vi "main.vi"() -> ()   [LabVIEW 2014]
uses:
  <vilib>/picture/3D Picture Control/Object/Create Object (drawable).vi
  <vilib>/picture/3D Picture Control/Object/Add Object (reference).vi
  <vilib>/Instr/_visa.llb/VISA Configure Serial Port (Instr).vi
  <vilib>/picture/3D Picture Control/NI_3D Picture Control.lvlib
panel:
  out "8号温度":i32
  out "7号温度":i32
  out "6号温度":i32
  out "未安装":dbl(slide) scale=0.0..5000.0
  out "未安装":dbl(slide) scale=0.0..5000.0
  out "6号温度":dbl(slide) scale=0.0..5000.0
  out "5号温度":dbl(slide) scale=0.0..5000.0
  out "4号温度":dbl(slide) scale=0.0..5000.0
  out "3号温度":dbl(slide) scale=0.0..5000.0
  out "2号温度":dbl(slide) scale=0.0..5000.0
  out "1号温度":dbl(slide) scale=0.0..5000.0
  out "?":T1(graph)
  out "5号温度":i32
  out "4号温度":i32
  out "2号温度":i32
  out "3号温度":i32
  out "1号温度":i32
  in  "停止":bool
  in  "打开":bool caption="stop"
  in  "校验位：":u16(ring) items=["  无校验", "  奇校验", "  偶校验"]
  in  "波特率：":u16(ring)=11 items=["   300", "   600", "   1200", "   2400", "   4800   ", "   9600", "   19200", "   38400", "   43000", "   56000", "   57600", "   115200"]
  in  "通讯口：":u16(ring) items=["   com1", "   com2", "   com3", "   com4", "   com5"]
  out "工作指示灯":bool
  # "TETRAELC--检测DEMO"
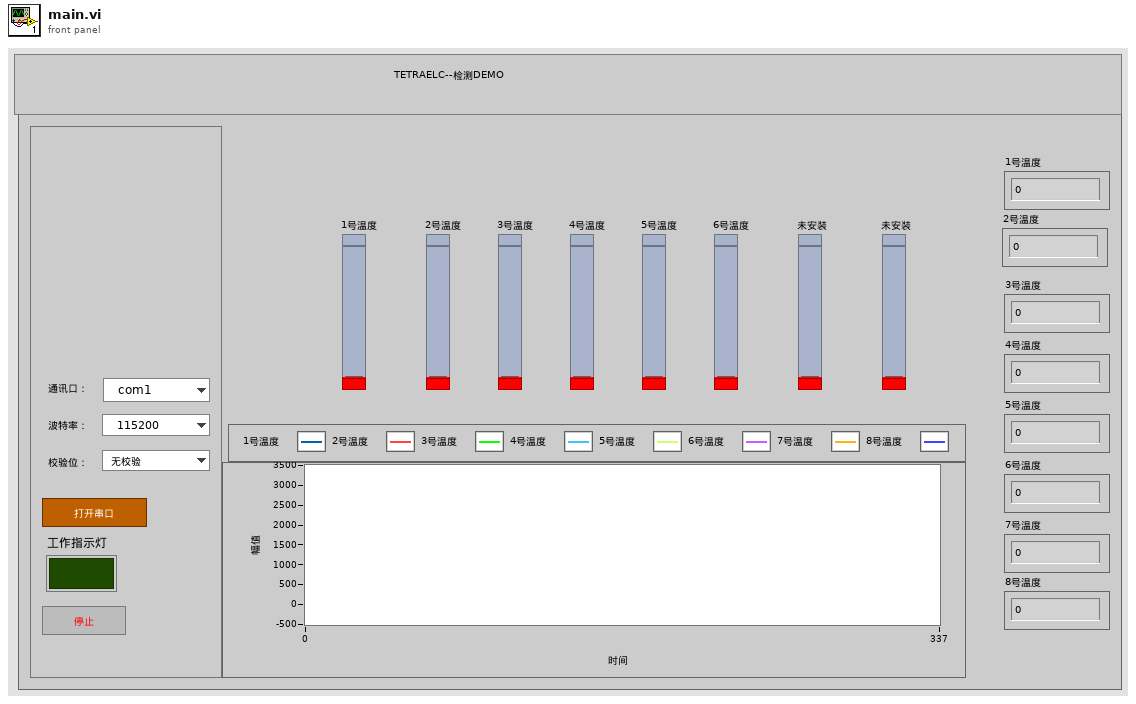
[diagram p1: front panel]
types:
  T1 = cluster{"1号温度":i32, "2号温度":i32, "3号温度":i32, "4号温度":i32, "5号温度":i32, "6号温度":i32, "7号温度":i32, "8号温度":i32}
  T2 = cluster{"T1":i16, "T2":i16, "T3":i16, "T4":i16, "T5":i16, "T6":i16, "T7":i16, "T8":i16}
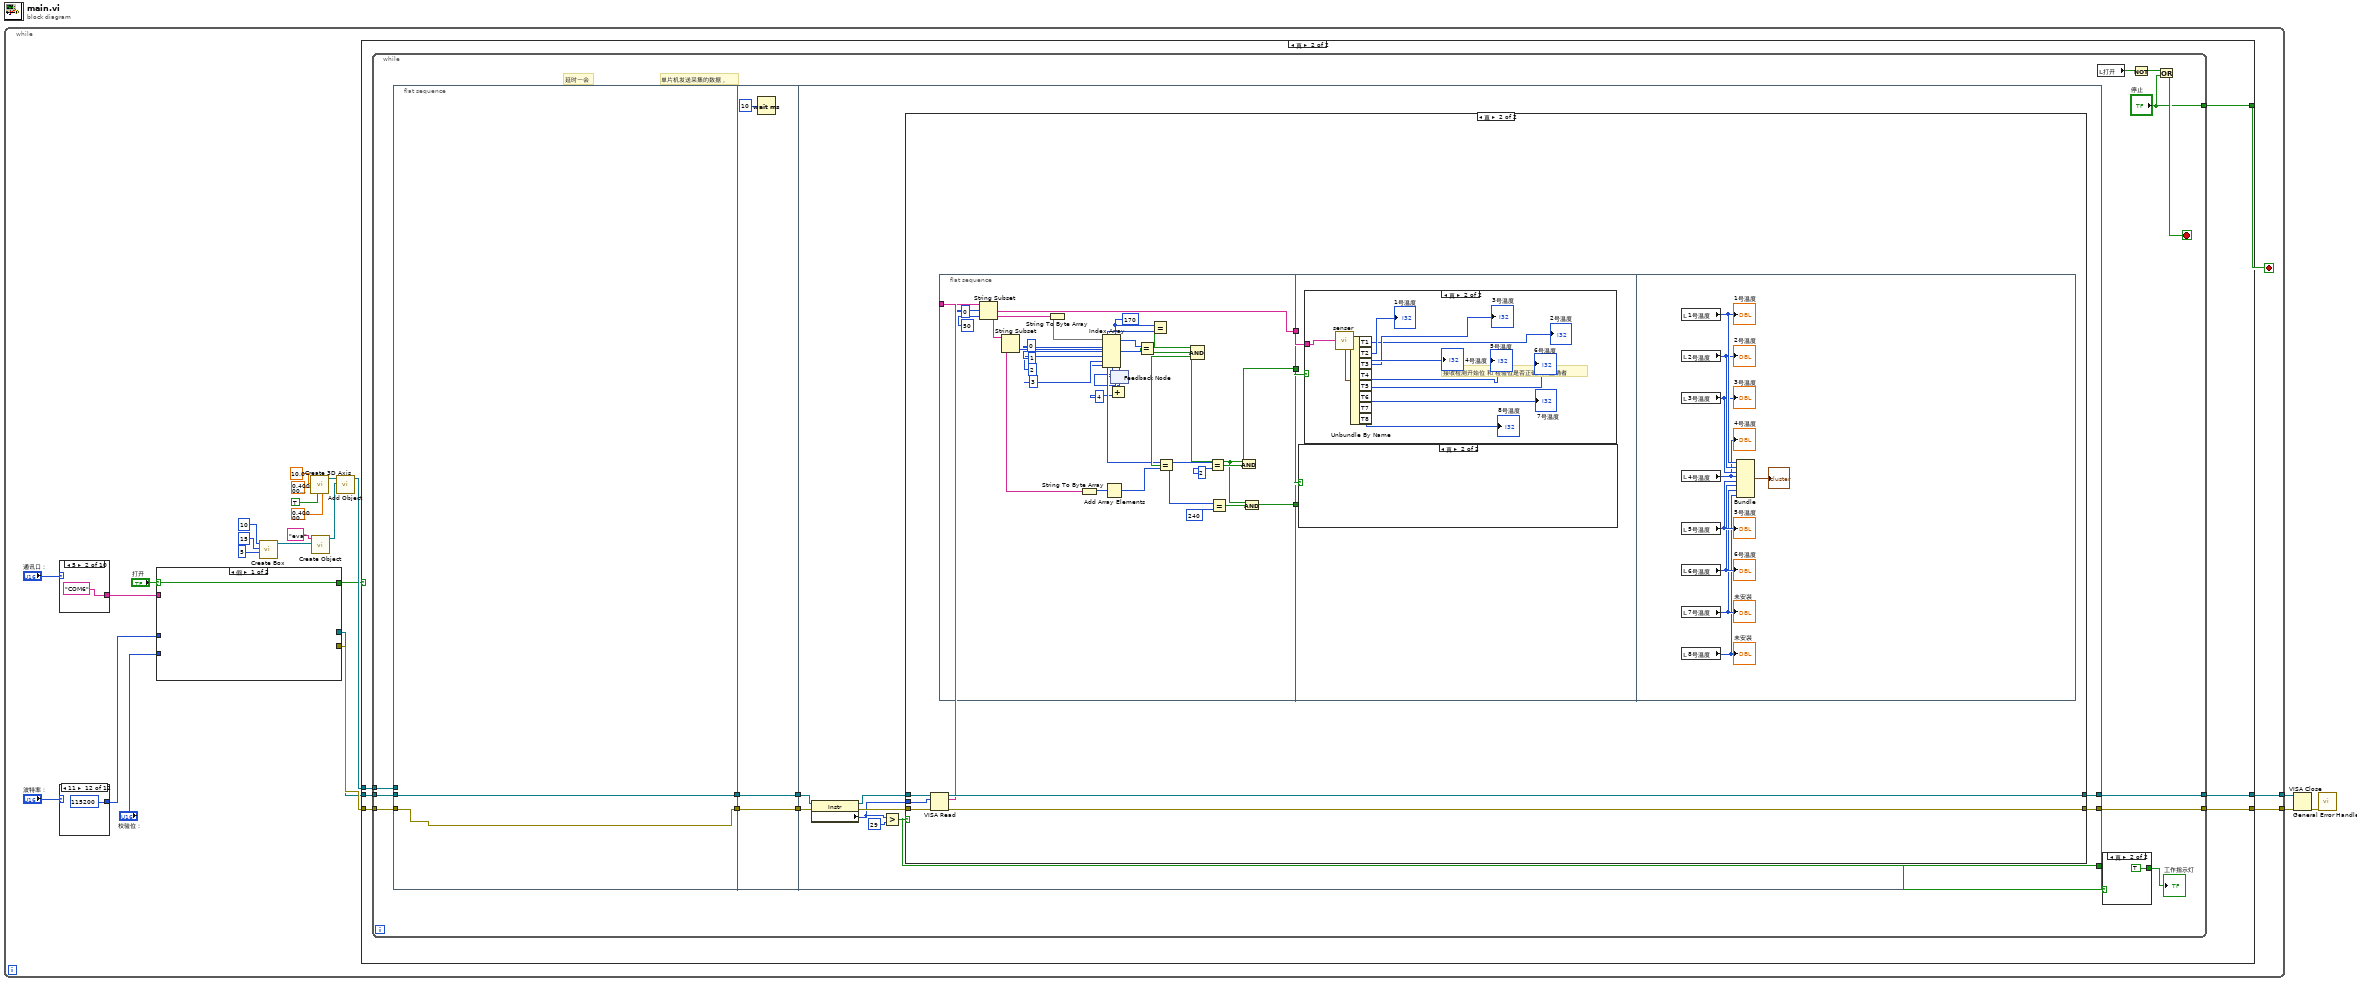
[diagram p0: block diagram]
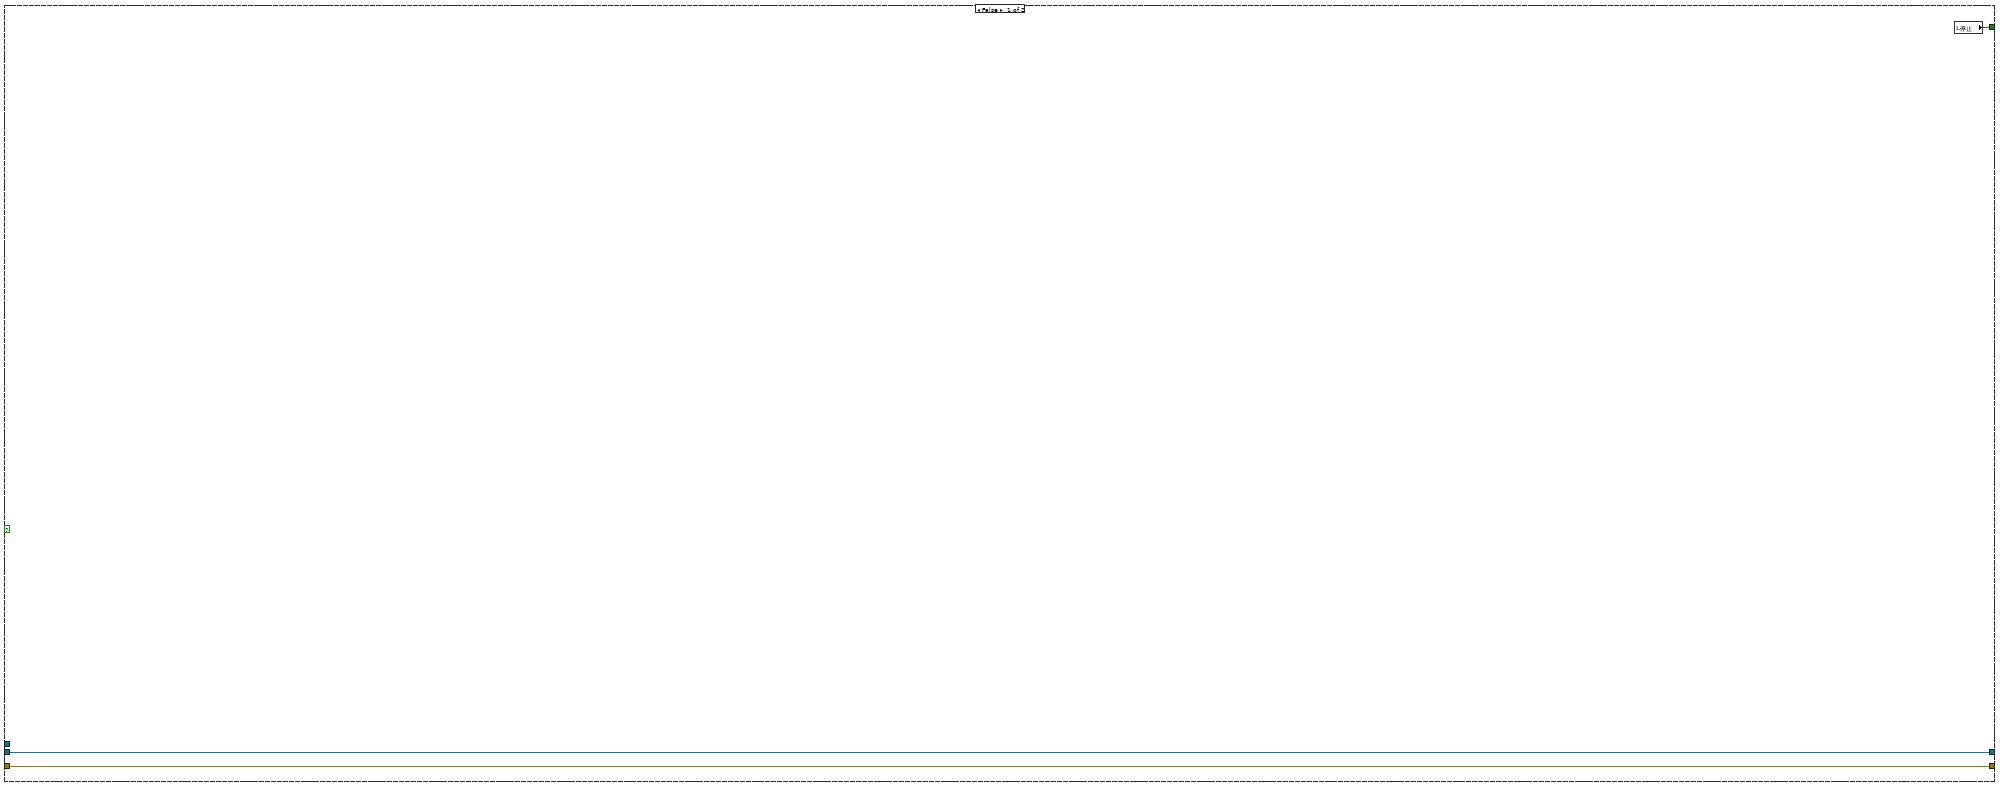
[diagram p2: hidden frame]
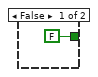
[diagram p3: hidden frame]
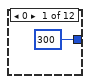
[diagram p7: hidden frame]
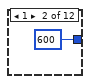
[diagram p8: hidden frame]
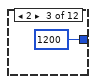
[diagram p9: hidden frame]
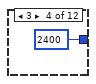
[diagram p10: hidden frame]
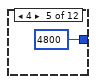
[diagram p11: hidden frame]
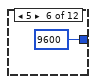
[diagram p12: hidden frame]
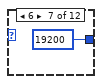
[diagram p13: hidden frame]
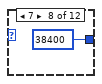
[diagram p14: hidden frame]
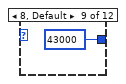
[diagram p15: hidden frame]
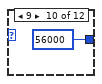
[diagram p16: hidden frame]
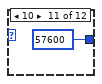
[diagram p17: hidden frame]
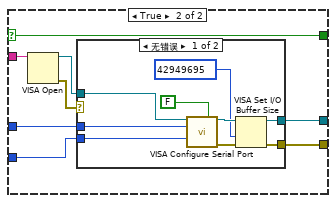
[diagram p18: hidden frame]
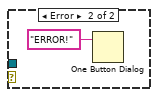
[diagram p19: hidden frame]
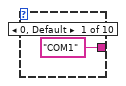
[diagram p20: hidden frame]
diagram:
  n1 = while {
    tunnel: [w26] -> w3
    tunnel: [w25] -> w2
    stop <- w5 stop-if-true
    n2 = case shown="5" "通讯口：" {
      tunnel: ["COM1" "COM6" "COM6" "COM2" "COM7" "COM3" "COM9" "COM8" "COM4" "COM5"] -> w9
      frame 0, Default {
      }
      frame 5 {
      }
      frame 6 {
      }
      frame 1 {
      }
      frame 7 {
      }
      frame 2 {
      }
      frame 9 {
      }
      frame 8 {
      }
      frame 3 {
      }
      frame 4 {
      }
    }
    n3 = case shown="11" "波特率：" {
      tunnel: [300 600 1200 2400 4800 9600 19200 38400 43000 56000 57600 115200] -> w6
      frame 0 {
      }
      frame 1 {
      }
      frame 2 {
      }
      frame 3 {
      }
      frame 4 {
      }
      frame 5 {
      }
      frame 6 {
      }
      frame 7 {
      }
      frame 8, Default {
      }
      frame 9 {
      }
      frame 10 {
      }
      frame 11 {
      }
    }
    n4 = case shown="假" "打开" {
      selector: "打开" -> [w144 w152]
      tunnel: w6 -> [_ w148]
      tunnel: [w144 w152] -> w4
      tunnel: [_ w146] -> w23
      tunnel: [_ w145] -> w27
      tunnel: w9 -> [_ w151]
      tunnel: "校验位：" -> [_ w147]
      frame False {
      }
      frame True {
        n5 = VISA Open(VISA resource name=w151) -> (VISA resource name=w149:refnum<visa-resource-name>, error out=w150:errorcluster)  [unwired: 4 in]
        n6 = case shown="无错误" w150 {
          tunnel: w149 -> [w161 _]
          tunnel: w148 -> [w160 _]
          tunnel: w147 -> [w159 _]
          tunnel: [w155 _] -> w146
          tunnel: [w156 _] -> w145
          frame No Error {
            n7 = call-poly "VISA Configure Serial Port"("VISA resource name"=w161, "Enable Termination\nChar (T)"=FALSE, "baud rate (9600)"=w160, "parity (0:none)"=w159) -> ("VISA resource name out"=w158:refnum<visa-resource-name>, "error out"=w157:errorcluster)  [unwired: 10 in]
            n8 = VISA Set I/O Buffer Size(VISA resource name=w158, size (4096)=u32 42949695 ("大小(4096)"), error in (no error)=w157) -> (VISA resource name out=w155:refnum<visa-resource-name>, error out=w156:errorcluster)  [unwired: 1 in]
          }
          frame Error {
            n9 = One Button Dialog(message="ERROR!" ("消息")) -> ()  [unwired: 1 in, 1 out]
          }
        }
      }
    }
    n10 = call <vilib>:"Create Box.vi"("Length Z"=5, "Length Y"=15, "Length X"=10) -> ("New Box Refnum"=w18:refnum<vi>)  [unwired: 7 in, 1 out]
    n11 = call <vilib>:"Create 3D Axis.vi"("Character Size"=sgl 0.4, "Axis label?"=TRUE, "Radius"=sgl 0.4, "Length"=sgl 10.0) -> ("New Object Refnum"=w12:refnum<vi>)  [unwired: 6 in, 1 out]
    n12 = call-poly <vilib>:"Create Object.vi"("Geometry"=w18, "Name"="eva") -> ("Scene:New Object"=w17:refnum<vi>)  [unwired: 8 in, 1 out]
    n13 = call-poly <vilib>:"Add Object.vi"("New Object In"=w17, "Scene Object In"=w12) -> ("Scene Object Out"=w24:refnum<vi>)  [unwired: 7 in, 2 out]
    n14 = case shown="真" w4 {
      tunnel: w27 -> [w28 w36]
      tunnel: [w29 w35] -> w26
      tunnel: [w28 w34] -> w25
      tunnel: w24 -> [_ w33]
      tunnel: w23 -> [w29 w32]
      tunnel: [w30 w31] -> w5
      frame False {
        n15 = local read "停止"() -> (w30:bool)
      }
      frame True {
        n16 = while {
          tunnel: w32 -> [w49]
          tunnel: w36 -> [w48]
          tunnel: [w47] -> w35
          tunnel: [w46] -> w34
          tunnel: w33 -> [w43]
          tunnel: ["停止"] -> w31
          stop <- w42 stop-if-true
          # "单片机发送采集的数据，"
          # "延时一会"
          n17 = flat-sequence {
            tunnel: w49 -> [w55]
            tunnel: w48 -> [w54]
            tunnel: w43 -> [_]
            tunnel: [w55] -> w38
            tunnel: [w54] -> w37
            tunnel: [w58] -> w51
            tunnel: [w57] -> w50
            tunnel: w38 -> [w58]
            tunnel: w37 -> [w57]
            tunnel: w51 -> [w66]
            tunnel: w50 -> [w65]
            tunnel: [w67] -> w46
            tunnel: [w62] -> w47
            tunnel: [w61] -> w44
            frame #0 {
            }
            frame #1 {
              n18 = Wait (ms)(milliseconds to wait=u32 10 ("等待时间（毫秒）")) -> ()  [unwired: 1 out]
            }
            frame #2 {
              n19 = property class="Instr"(reference=w66, error in=w65) -> (reference out=w64:refnum<visa-resource-name>, error out=w63:errorcluster, "Serial Settings:Number of Bytes at Serial Port"=w60:u32)
              n20 = Greater?(x=w60, y=u32 29) -> (0:w61:bool)
              n21 = case shown="真" w61 {
                tunnel: [w68 w71] -> w67
                tunnel: w64 -> [w69 w78]
                tunnel: w63 -> [w68 w72]
                tunnel: [w69 w77] -> w62
                tunnel: w60 -> [_ w76]
                frame False {
                }
                frame True {
                  n22 = VISA Read(VISA resource name=w78, byte count=w76, error in (no error)=w72) -> (VISA resource name out=w77:refnum<visa-resource-name>, read buffer=w75:string, error out=w71:errorcluster)  [unwired: 1 out]
                  n23 = flat-sequence {
                    tunnel: w75 -> [w101]
                    tunnel: [w100] -> w74
                    tunnel: [w80] -> w73
                    tunnel: [w79] -> w70
                    tunnel: w74 -> [w112]
                    tunnel: w73 -> [w111]
                    tunnel: w70 -> [w110]
                    frame #0 {
                      w99 = 170 ("长度（剩余）")
                      n24 = String Subset(string=w101, offset (0)=0 ("长度（剩余）"), length (rest)=50 ("长度（剩余）")) -> (substring=w100:string)
                      n25 = String To Byte Array(string=w100) -> (unsigned byte array=w109:u8[])
                      n26 = feedback #1() -> (w82:u8)  [unwired: 1 in]
                      n27 = Index Array(array=w109, index #1=0 ("长度（剩余）"), index #2=1 ("长度（剩余）"), index #3=2 ("索引"), index #4=3 ("索引"), index #5=w82) -> (element #1=w108:u8, element #2=w98:u8, element #3=w90:u8, element #4=w84:u8, element #5=w92:u8)
                      n28 = Add(x=w84, y=u8 4) -> (x+y=w81:u8)
                      n29 = String Subset(string=w100, length (rest)=w81) -> (substring=w102:string)  [unwired: 1 in]
                      n30 = String To Byte Array(string=w102) -> (unsigned byte array=w104:u8[])
                      n31 = Add Array Elements(numeric array=w104) -> (sum=w83:u8)
                      n32 = feedback-in #1(w81) -> ()
                      n33 = Equal?(x=w99, y=w98) -> (x = y?=w95:bool)
                      n34 = Equal?(x=w99, y=w108) -> (x = y?=w96:bool)
                      n35 = Equal?(x=w92, y=w83) -> (x = y?=w94:bool)
                      n36 = Compound Arithmetic op=AND(w96, w95, w94) -> (w85:bool)
                      n37 = Equal?(x=w90, y=u8 2) -> (x = y?=w87:bool)
                      n38 = Equal?(x=w90, y=u8 240) -> (x = y?=w86:bool)
                      n39 = And(x=w85, y=w87) -> (x .and. y?=w80:bool)
                      n40 = And(x=w85, y=w86) -> (x .and. y?=w79:bool)
                    }
                    frame #1 {
                      n41 = case shown="真" w110 {
                        frame False {
                        }
                        frame True {
                        }
                      }
                      n42 = case shown="真" w111 {
                        tunnel: w112 -> [_ w122]
                        frame False {
                        }
                        frame True {
                          # "接收检测开始位 和 检验位是否正确如果正确者"
                          n43 = call "senser.vi"("read buffer"=w122) -> ("输出簇"=w121:T2)
                          n44 = Unbundle By Name(w121) -> ("T1"=→"2号温度":i16, "T2"=→"1号温度":i16, "T3"=→"3号温度":i16, "T4"=→"4号温度":i16, "T5"=→"5号温度":i16, "T6"=→"6号温度":i16, "T7"=→"7号温度":i16, "T8"=→"8号温度":i16)
                        }
                      }
                    }
                    frame #2 {
                      n45 = local read "1号温度"() -> (w130:i32)
                      "1号温度" <- w130
                      n46 = local read "2号温度"() -> (w129:i32)
                      "2号温度" <- w129
                      n47 = local read "3号温度"() -> (w128:i32)
                      "3号温度" <- w128
                      n48 = local read "4号温度"() -> (w127:i32)
                      "4号温度" <- w127
                      n49 = local read "5号温度"() -> (w126:i32)
                      "5号温度" <- w126
                      n50 = local read "6号温度"() -> (w125:i32)
                      "6号温度" <- w125
                      n51 = local read "7号温度"() -> (w124:i32)
                      "未安装" <- w124
                      n52 = local read "8号温度"() -> (w123:i32)
                      "未安装" <- w123
                      n53 = Bundle("1号温度"=w130, "2号温度"=w129, "3号温度"=w128, "4号温度"=w127, "5号温度"=w126, "6号温度"=w125, "7号温度"=w124, "8号温度"=w123) -> (→"?":T1)  [unwired: 1 in]
                    }
                  }
                }
              }
            }
          }
          n54 = local read "打开"() -> (w40:bool)
          n55 = case shown="真" w44 {
            tunnel: [FALSE ("工作指示灯") TRUE ("工作指示灯")] -> w45
            frame False {
            }
            frame True {
            }
          }
          "工作指示灯" <- w45
          n56 = Not(x=w40) -> (.not. x?=w41:bool)
          n57 = Or(x=w41, y="停止") -> (x .or. y?=w42:bool)
        }
      }
    }
  }
  n58 = VISA Close(VISA resource name=w3, error in (no error)=w2) -> (error out=w1:errorcluster)
  n59 = call <vilib>:"General Error Handler.vi"("error in (no error)"=w1) -> ()  [unwired: 10 in, 5 out]
